vi "Drive - Joystick Set.vi"(8 "error in (no error)":errorcluster, 11 "Axes":dbl[](array[numeric])) -> (0 "error out":errorcluster, 1 "gain":dbl(slide) scale=-1.0..1.0, 2 "r":dbl(slide) scale=-1.0..1.0, 3 "l":dbl(slide) scale=-1.0..1.0)   [LabVIEW 2014]
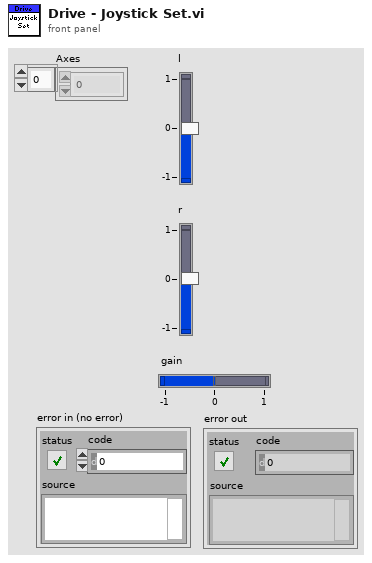
[diagram p1: front panel]
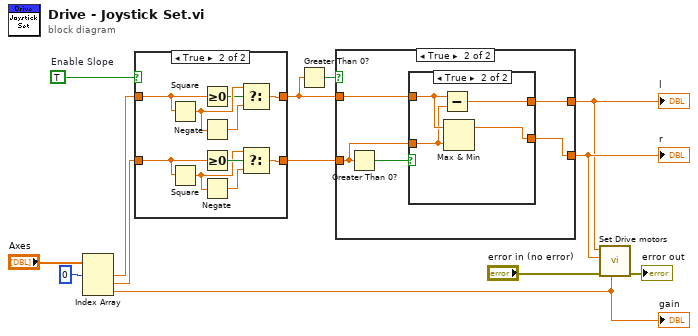
[diagram p0: block diagram]
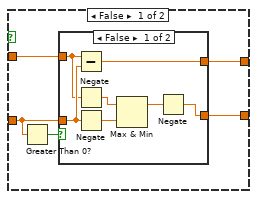
[diagram p3: hidden frame]
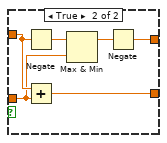
[diagram p4: hidden frame]
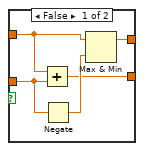
[diagram p5: hidden frame]
diagram:
  w6 = TRUE  # Enable Slope
  n1 = Index Array(array="Axes", index #1=0) -> (element #1=w5:dbl, element #2=w10:dbl, element #3=w11:dbl)  [unwired: 2 in]
  "gain" <- w11
  n2 = case shown="True" w6 {
    tunnel: [w14 w25] -> w8
    tunnel: [w15 w24] -> w7
    tunnel: w10 -> [w14 w23]
    tunnel: w5 -> [w15 w22]
    frame False {
    }
    frame True {
      n3 = Square(x=w22) -> (x^2=w17:dbl)
      n4 = Square(x=w23) -> (x^2=w20:dbl)
      n5 = Greater Or Equal To 0?(x=w22) -> (x >= 0?=w16:bool)
      n6 = Negate(x=w17) -> (-x=w18:dbl)
      n7 = Greater Or Equal To 0?(x=w23) -> (x >= 0?=w21:bool)
      n8 = Negate(x=w20) -> (-x=w19:dbl)
      n9 = Select(t=w17, s=w16, f=w18) -> (s? t:f=w24:dbl)
      n10 = Select(t=w20, s=w21, f=w19) -> (s? t:f=w25:dbl)
    }
  }
  n11 = Greater Than 0?(x=w7) -> (x > 0?=w4:bool)
  n12 = case shown="True" w4 {
    tunnel: w8 -> [w29 w47]
    tunnel: w7 -> [w28 w46]
    tunnel: [w27 w45] -> w12
    tunnel: [w26 w44] -> w13
    frame False {
      n13 = Greater Than 0?(x=w29) -> (x > 0?=w30:bool)
      n14 = case shown="False" w30 {
        tunnel: w29 -> [w37 w39]
        tunnel: w28 -> [w35 w40]
        tunnel: [w31 w41] -> w27
        tunnel: [w32 w38] -> w26
        frame False {
          n15 = Subtract(x=w35, y=w37) -> (x-y=w31:dbl)
          n16 = Negate(x=w35) -> (-x=w36:dbl)
          n17 = Negate(x=w37) -> (-x=w34:dbl)
          n18 = Max & Min(x=w36, y=w34) -> (max(x,y)=w33:dbl)  [unwired: 1 out]
          n19 = Negate(x=w33) -> (-x=w32:dbl)
        }
        frame True {
          n20 = Negate(x=w40) -> (-x=w43:dbl)
          n21 = Add(x=w40, y=w39) -> (x+y=w38:dbl)
          n22 = Max & Min(x=w43, y=w39) -> (max(x,y)=w42:dbl)  [unwired: 1 out]
          n23 = Negate(x=w42) -> (-x=w41:dbl)
        }
      }
    }
    frame True {
      n24 = Greater Than 0?(x=w47) -> (x > 0?=w48:bool)
      n25 = case shown="True" w48 {
        tunnel: w47 -> [w53 w55]
        tunnel: w46 -> [w50 w56]
        tunnel: [w51 w54] -> w45
        tunnel: [w49 w57] -> w44
        frame False {
          n26 = Add(x=w50, y=w53) -> (x+y=w49:dbl)
          n27 = Negate(x=w53) -> (-x=w52:dbl)
          n28 = Max & Min(x=w50, y=w52) -> (max(x,y)=w51:dbl)  [unwired: 1 out]
        }
        frame True {
          n29 = Subtract(x=w56, y=w55) -> (x-y=w54:dbl)
          n30 = Max & Min(x=w56, y=w55) -> (max(x,y)=w57:dbl)  [unwired: 1 out]
        }
      }
    }
  }
  "r" <- w13
  "l" <- w12
  n31 = call "Set Drive motors.vi"("Gain"=w11, "error in (no error)"="error in (no error)", "Right"=w13, "Left"=w12) -> ("error out"=→"error out":errorcluster)  [unwired: 7 in]
